vi "ReadSlideImage.vi"(1 "file name":string, 2 "Full Size":bool=TRUE) -> (0 "Image":T1 {"Dialogs" format="%.0b"})   [LabVIEW 2012]
uses:
  <userlib>/ImageProcessing/QTLIB_2595_LV86/QT_Image.ctl
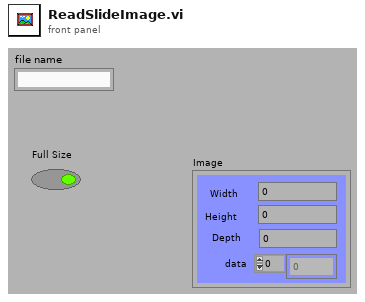
[diagram p1: front panel]
types:
  T1 = typedef "QT_Image.ctl" = cluster{"Width":i32, "Height":i32, "Depth":i32, "data":u8[], "Compressed data":u8[], "Color table":u32[], "Duration":i32, "Options":i32, "Timestamp":i32, "ID":i32, "Reserved":i32, "Dialogs":u32}
  T2 = typedef "imagedata.ctl" = cluster{"image type":i32, "image depth":i32, "image":u8[], "mask":u8[], "colors":u32[], "Rectangle":cluster{"left":i16, "top":i16, "right":i16, "bottom":i16}}
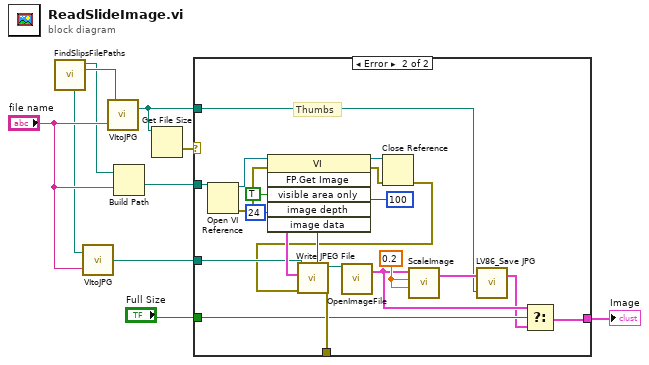
[diagram p0: block diagram]
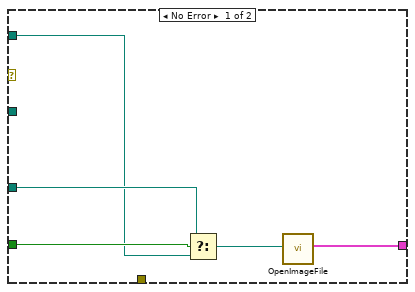
[diagram p2: hidden frame]
diagram:
  n1 = call "FindSlipsFilePaths.vi"() -> ("Images"=w3:path, "Thumbs"=w5:path, "Slides"=w2:path)  [unwired: 2 in, 2 out]
  n2 = call "VItoJPG.vi"("name"="file name", "Dest"=w3) -> ("appended path"=w6:path)
  n3 = call "VItoJPG.vi"("name"="file name", "Dest"=w5) -> ("appended path"=w9:path)
  n4 = Build Path(base path=w2, name or relative path="file name") -> (appended path=w1:path)
  n5 = Get File Size(file=w9) -> (0:w8:errorcluster)  [unwired: 1 in, 2 out]
  n6 = case shown="Error" w8 {
    tunnel: w9 -> [w12 w21]
    tunnel: w1 -> [_ w35]
    tunnel: [_ w26] -> _
    tunnel: w6 -> [w13 w22]
    tunnel: [w15 w16] -> w10
    tunnel: "Full Size" -> [w14 w19]
    frame No Error {
      n7 = Select(t=w13, s=w14, f=w12) -> (s? t:f=w11:path)
      n8 = call <userlib>:"OpenImageFile.vi"("selected path"=w11) -> ("Image Out"=w15:T1)  [unwired: 2 in]
    }
    frame Error {
      w24 = 0.2 ("X scale")
      # "Thumbs"
      n9 = Open VI Reference(vi path=w35) -> (vi reference=w34:refnum<vi>, error out=w33:errorcluster)  [unwired: 5 in]
      n10 = invoke class="VI" method="FP.Get Image"(reference=w34, error in=w33, "visible area only"=TRUE ("Visible Area Only"), "image depth"=24 ("Image Depth")) -> (reference out=w29:refnum<vi>, error out=w30:errorcluster, "image data"=w28:T2)  [unwired: 2 in, 3 out]
      n11 = Close Reference(reference=w29, error in (no error)=w30) -> (error out=w20:errorcluster)
      n12 = call <vilib>:"Write JPEG File.vi"("quality (80)"=100, "error in (no error)"=w20, "image data"=w28, "path to JPEG file"=w22) -> ("error out"=w26:errorcluster, "path"=w25:path)  [unwired: 6 in]
      n13 = call <userlib>:"OpenImageFile.vi"("selected path"=w25) -> ("Image Out"=w18:T1)  [unwired: 2 in]
      n14 = call <userlib>:"ScaleImage.vi"("X scale"=w24, "Y scale"=w24, "Image in"=w18) -> ("Image Out"=w23:T1)  [unwired: 2 in]
      n15 = call <userlib>:"LV86_Save JPG.vi"("Path to file"=w21, "Image"=w23) -> ("Image"=w17:T1)  [unwired: 1 in]
      n16 = Select(t=w18, s=w19, f=w17) -> (s? t:f=w16:T1)
    }
  }
  "Image" <- w10
